vi "Enq Msg.vi"(6 "우선순위 메시지?":bool, 8 "에러 입력(에러 없음)":errorcluster, 9 "값":variant, 10 "메세지":string, 11 "큐 입력":refnum<queue>) -> (0 "에러 출력":errorcluster, 3 "큐 출력":refnum<queue>)   [LabVIEW 2020]
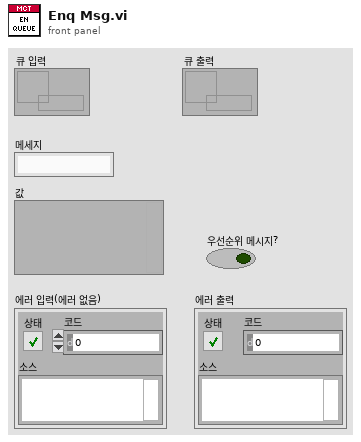
[diagram p1: front panel]
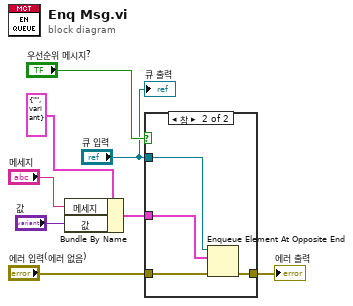
[diagram p0: block diagram]
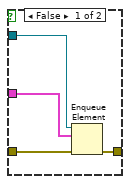
[diagram p2: hidden frame]
diagram:
  n1 = Bundle By Name(cluster=cluster{"메세지":string, "값":variant} {"메세지"="", "값"=variant} ("원소"), "메세지"="메세지", "값"="값") -> (w5:cluster{"메세지":string, "값":variant})
  n2 = case shown="참" "우선순위 메시지?" {
    tunnel: "큐 입력" -> [w12 w16]
    tunnel: [w11 w15] -> w2
    tunnel: "에러 입력(에러 없음)" -> [w10 w14]
    tunnel: w5 -> [w9 w13]
    frame False {
      n3 = Enqueue Element(queue=w12, element=w9, error in (no error)=w10) -> (error out=w11:errorcluster)  [unwired: 1 in, 2 out]
    }
    frame True {
      n4 = Enqueue Element At Opposite End(queue=w16, element=w13, error in (no error)=w14) -> (error out=w15:errorcluster)  [unwired: 1 in, 2 out]
    }
  }
  "에러 출력" <- w2
  "큐 출력" <- "큐 입력"
